vi "Destroy.vi"(0 "reference in":refnum<class "Items Controller.lvclass">, 5 "error in (no error)":errorcluster) -> (14 "reference out":refnum<class "Items Controller.lvclass">, 19 "error out":errorcluster)   [LabVIEW 2014, in "Items Controller.lvclass"]
doc: "Destructor."
uses:
  Items Controller.lvclass
  <vilib>/addons/_AddQ/G#Object/G#Object.lvclass
  APP/checkIN_class/checkIN.lvclass
  APP/checkOUT_class/checkOUT.lvclass
  APP/item_class/item.lvclass
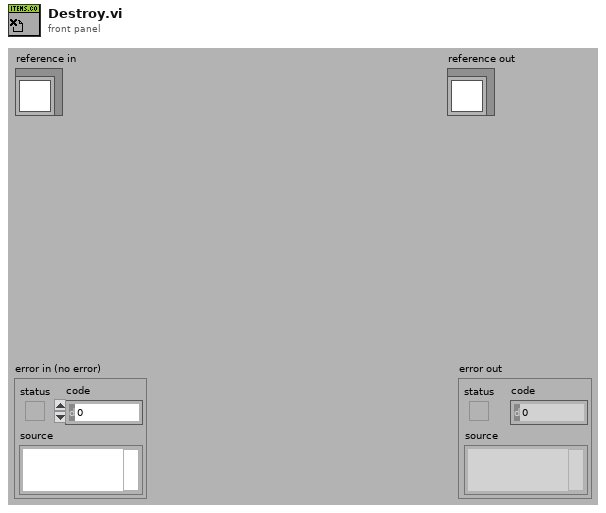
[diagram p1: front panel]
types:
  T1 = typedef "Items Controller.lvclass/ObjectAttributes.ctl" = cluster{"MyAttribute":dbl, "data":string[][][], "file_controller_ref":refnum<class "File Controller.lvclass">, "checkIN_ref":refnum<class "checkIN.lvclass">, "checkOUT_ref":refnum<class "checkOUT.lvclass">, "item_ref":refnum<class "item.lvclass">}
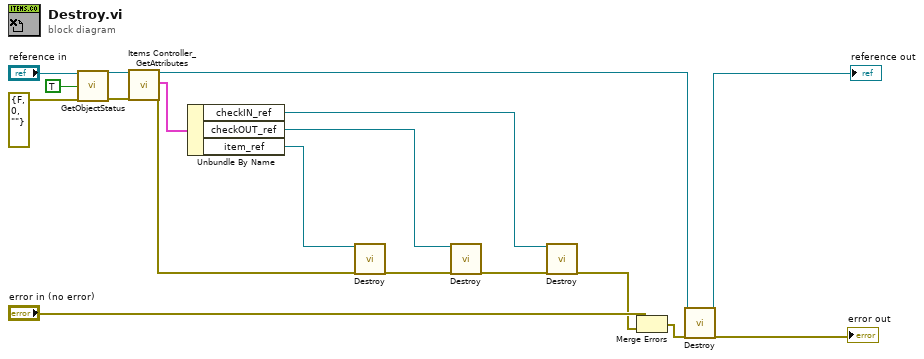
[diagram p0: block diagram]
diagram:
  n1 = call-dynamic "GetObjectStatus.vi"("reference in"="reference in", "simple info (F)"=TRUE ("simple info"), "error in (no error)"=errorcluster {"status"=FALSE, "code"=0, "source"=""}) -> ("reference out"=w12:refnum<class "Items Controller.lvclass">, "error out"=w13:errorcluster)  [unwired: 5 in, 10 out]
  n2 = call "Items Controller_GetAttributes.vi"("reference in"=w12, "error in (no error)"=w13) -> ("reference out"=w11:refnum<class "Items Controller.lvclass">, "attributes"=w10:T1, "error out"=w6:errorcluster)  [unwired: 14 in, 1 out]
  n3 = Unbundle By Name(w10) -> ("checkIN_ref"=w1:refnum<class "checkIN.lvclass">, "checkOUT_ref"=w5:refnum<class "checkOUT.lvclass">, "item_ref"=w7:refnum<class "item.lvclass">)
  n4 = call-dynamic "Destroy.vi"("reference in"=w7, "error in (no error)"=w6) -> ("error out"=w4:errorcluster)  [unwired: 16 in, 1 out]
  n5 = call-dynamic "Destroy.vi"("reference in"=w5, "error in (no error)"=w4) -> ("error out"=w3:errorcluster)  [unwired: 16 in, 1 out]
  n6 = call-dynamic "Destroy.vi"("reference in"=w1, "error in (no error)"=w3) -> ("error out"=w2:errorcluster)  [unwired: 16 in, 1 out]
  n7 = Merge Errors("error in (no error)", w2) -> (w17:errorcluster)
  n8 = call-parent "Destroy.vi"("reference in"=w11, "error in (no error)"=w17) -> ("reference out"=→"reference out":refnum<class "Items Controller.lvclass">, "error out"=→"error out":errorcluster)  [unwired: 16 in]
